vi "XNET String To IO Name (Session).vi"(3 "string":string) -> (0 "XNET Session":refnum<k21>)   [LabVIEW 2018]
doc: "Converts a LabVIEW string to an XNET Session I/O name."
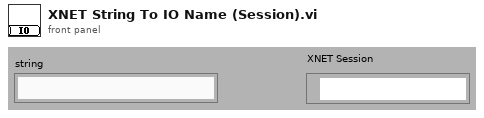
[diagram p1: front panel]
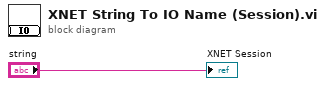
[diagram p0: block diagram]
diagram:
  "XNET Session" <- "string"
